vi "Global.vi"() -> ()   [LabVIEW 2013]
panel:
  out "ActCtl":bool[](array[boolean])
  in  "COM":T1
  out "Log":refnum<user-event>
  out "Result":refnum<user-event>
  in  "同步启动个数":u8=8 min=1 max=8 step=1
  in  "测试方式":enum16{"震动前测试", "震动测试"}(ring)
  in  "Stop":bool
  in  "Exit":bool
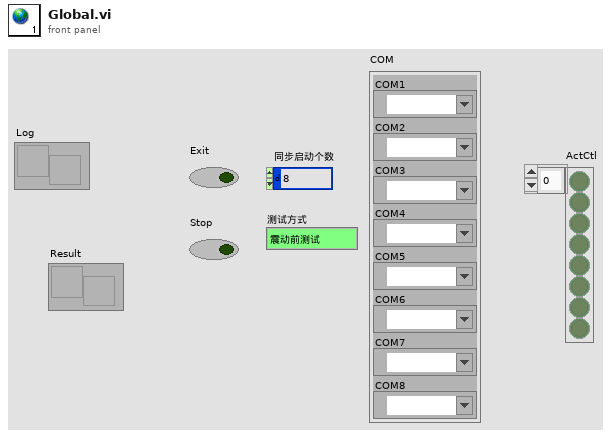
[diagram p1: front panel]
types:
  T1 = cluster{"COM1":refnum<visa-resource-name>, "COM2":refnum<visa-resource-name>, "COM3":refnum<visa-resource-name>, "COM4":refnum<visa-resource-name>, "COM5":refnum<visa-resource-name>, "COM6":refnum<visa-resource-name>, "COM7":refnum<visa-resource-name>, "COM8":refnum<visa-resource-name>}
diagram:
